vi "Mouse Down Valid.vi"(8 "error in (no error)":errorcluster, 9 "Mods":cluster{"Double Click":bool, "Menu Key":bool}, 10 "Coords":cluster{"Horizontal":i32, "Vertical":i32}, 11 "UI_Top_Customer in":refnum<class "UI_Top_Customer.lvclass">) -> (0 "error out":errorcluster, 3 "UI_Top_Customer out":refnum<class "UI_Top_Customer.lvclass">)   [LabVIEW 2021, in "UI_Top_Customer.lvclass"]
uses:
  UI_Top_Customer.lvclass
  UI_Top_Customer.lvclass/UI_Top_Customer.ctl
  <userlib>/John_Lib/Queue_Self/Queue_Self.lvlib
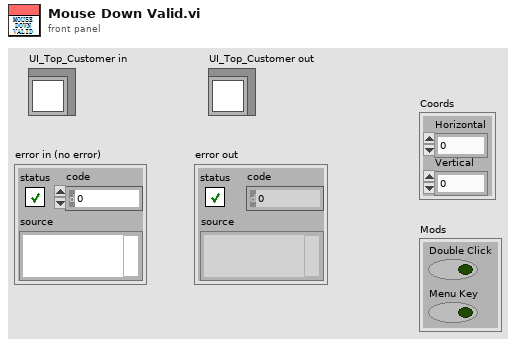
[diagram p1: front panel]
types:
  T1 = typedef "LVRectTypeDef.ctl" = cluster{"Left":i16, "Top":i16, "Right":i16, "Bottom":i16}
  T2 = typedef "UI_Top_Customer.lvclass/Pane MouseDown.ctl" = cluster{"Type":T3, "Coords":cluster{"Horizontal":i32, "Vertical":i32}, "Mods":cluster{"Double Click":bool, "Menu Key":bool}, "Pane: MouseDown":bool}
  T3 = typedef "lveventtype.ctl" = enum32{"Null", "Timeout", "Annotation Menu Selection", "Annotation Menu Selection?", "App Instance Close", "App Instance Close?", "Autoscale Range Change", "Bookmark Info Change", "Cell Edit", "Cell Edit?", "Cursor Grab", "Cursor Grab?", "Cursor Menu Selection", "Cursor Menu Selection?", "Cursor Move", "Cursor Release", "Data Change", "Direction Change", "Display State Change", "Drag Ended", "Drag Enter", "Drag Leave", "Drag Over", "Drag Source Update", "Drag Starting", "Drag Starting?", "Drop", "Exec State Change", "Key Down", "Key Down?", "Key Repeat", "Key Repeat?", "Key Up", "Listbox Double Click", "Menu Activation?", "Menu Selection (App)", "Menu Selection? (App)", "Menu Selection (User)", "Mouse Down", "Mouse Down?", "Mouse Enter", "Mouse Leave", "Mouse Move", "Mouse Up", "Mouse Wheel", "NI Security User Change (App)", "Pane Size", "Panel Close", "Panel Close?", "Panel Resize", "Plot Attribute Change", "Scale Range Change", "Shortcut Menu Activation?", "Shortcut Menu Selection (App)", "Shortcut Menu Selection? (App)", "Shortcut Menu Selection (User)", "Tree Double Click", "Tree Drag", "Tree Drag?", "Tree Drop", "Tree Drop?", "Tree Item Close", "Tree Item Close?", "Tree Item Open", "Tree Item Open?", "User Event", "Value Change"}
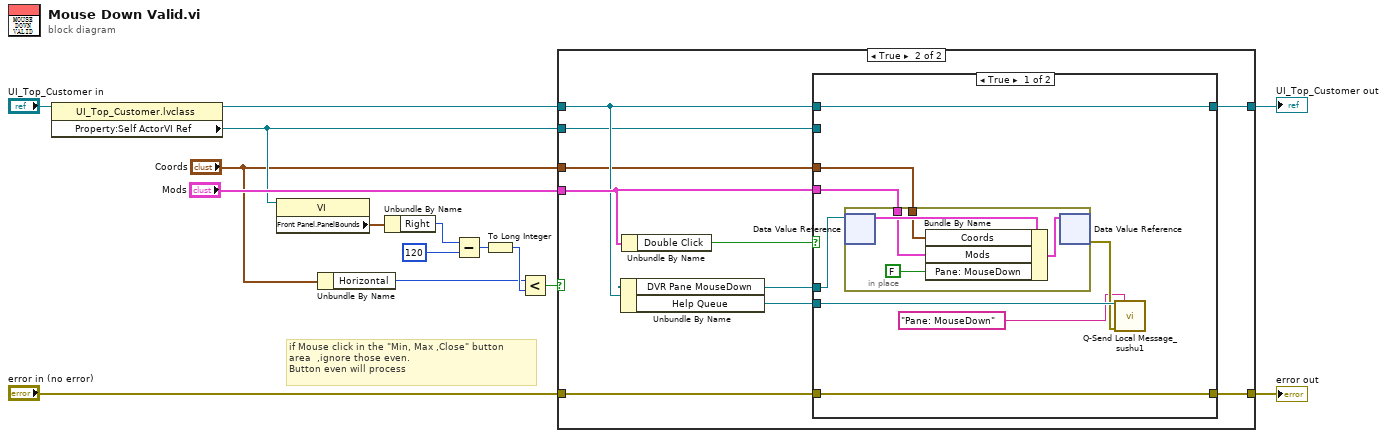
[diagram p0: block diagram]
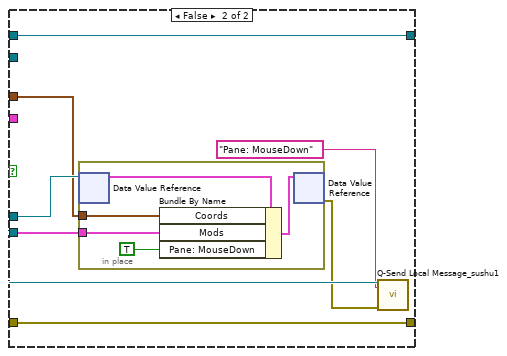
[diagram p3: hidden frame]
diagram:
  # "if Mouse click in the \"Min, Max ,Close\" button \narea  ,ignore those even.\nButton even will process"
  n1 = property class="UI_Top_Customer.lvclass"(reference="UI_Top_Customer in") -> (reference out=w13:refnum<class "UI_Top_Customer.lvclass">, "Property:Self ActorVI Ref"=w3:refnum<vi>)  [unwired: 1 in, 1 out]
  n2 = property class="VI"(reference=w3) -> ("Front Panel.PanelBounds"=w4:T1)  [unwired: 1 in, 2 out]
  n3 = Unbundle By Name("Coords") -> ("Horizontal"=w7:i32)
  n4 = Unbundle By Name(w4) -> ("Right"=w5:i16)
  n5 = Subtract(x=w5, y=i16 120) -> (x-y=w8:i16)
  n6 = To Long Integer(number=w8) -> (32bit integer=w9:i32)
  n7 = Less?(x=w7, y=w9) -> (x < y?=w1:bool)
  n8 = case shown="True" w1 {
    tunnel: "Mods" -> [_ w24]
    tunnel: w13 -> [w17 w23]
    tunnel: [w17 w22] -> w12
    tunnel: [w16 w21] -> w11
    tunnel: "error in (no error)" -> [w16 w20]
    tunnel: w3 -> [_ w19]
    tunnel: "Coords" -> [_ w18]
    frame False {
    }
    frame True {
      n9 = Unbundle By Name(w23) -> ("DVR Pane MouseDown"=w26:refnum<data-value>, "Help Queue"=w25:refnum<queue>)
      n10 = Unbundle By Name(w24) -> ("Double Click"=w27:bool)
      n11 = case shown="True" w27 {
        tunnel: w18 -> [w33 w43]
        tunnel: w24 -> [w32 w46]
        tunnel: w25 -> [w35 w48]
        tunnel: w26 -> [w34 w47]
        tunnel: w23 -> [w29 w45]
        tunnel: [w29 w45] -> w22
        tunnel: w19 -> [_ _]
        tunnel: [w28 w44] -> w21
        tunnel: w20 -> [w28 w44]
        frame True {
          n12 = in-place {
            in-place-border: w33 -> [w38]
            in-place-border: w32 -> [w37]
            n13 = in-place-dvr #1(w34) -> (w40:T2)  [unwired: 1 out]
            n14 = Bundle By Name(cluster=w40, "Coords"=w38, "Mods"=w37, "Pane: MouseDown"=FALSE) -> (w39:T2)
            n15 = in-place-dvr #1(w39) -> (w31:errorcluster)  [unwired: 1 out]
          }
          n16 = call <userlib>:"Q-Send Local Message_sushu1.vi"("queue in"=w35, "Elements in Front"="Pane: MouseDown", "error in"=w31) -> ()  [unwired: 10 in, 3 out]
        }
        frame False {
          n17 = in-place {
            in-place-border: w43 -> [w51]
            in-place-border: w46 -> [w50]
            n18 = in-place-dvr #2(w47) -> (w53:T2)  [unwired: 1 out]
            n19 = Bundle By Name(cluster=w53, "Coords"=w51, "Mods"=w50, "Pane: MouseDown"=TRUE) -> (w52:T2)
            n20 = in-place-dvr #2(w52) -> (w42:errorcluster)  [unwired: 1 out]
          }
          n21 = call <userlib>:"Q-Send Local Message_sushu1.vi"("queue in"=w48, "Elements in Front"="Pane: MouseDown", "error in"=w42) -> ()  [unwired: 10 in, 3 out]
        }
      }
    }
  }
  "error out" <- w11
  "UI_Top_Customer out" <- w12
